vi "Servo.vi"(8 "error in (no error)":errorcluster, 9 "Slow":bool, 10 "Function":T1, 11 "Servo":tag) -> (0 "error out":errorcluster)   [LabVIEW 2014]
uses:
  Controls/Conveyor Belt Functions.ctl
  <vilib>/myRIO/Common/Instrument Driver Framework/myRIO v1.0/PWM/vis/myRIO v1.1 Open PWM.vi
  <vilib>/myRIO/Common/Instrument Driver Framework/Utilities/vis/Validate Channels.vi
  <vilib>/myRIO/Common/Instrument Driver Framework/myRIO v1.0/PWM/vis/myRIO v1.0 Reserve PWM.vi
  <vilib>/myRIO/Common/Instrument Driver Framework/myRIO v1.0/PWM/vis/myRIO v1.0 Build MUX Configuration PWM.vi
  <vilib>/myRIO/Common/Instrument Driver Framework/myRIO v1.0/Resource Manager/vis/myRIO v1.0 Reserve Channel List.vi
  <vilib>/myRIO/Common/Instrument Driver Framework/myRIO v1.0/Resource Manager/vis/myRIO v1.0 Create Configuration List.vi
  <vilib>/myRIO/Common/Instrument Driver Framework/myRIO v1.0/Resource Manager/vis/myRIO v1.0 Reserve Channel.vi
  <vilib>/myRIO/Common/Instrument Driver Framework/myRIO v1.0/Resource Manager/vis/myRIO v1.0 Unreserve Channel.vi
  <vilib>/myRIO/Common/Instrument Driver Framework/myRIO v1.0/Resource Manager/vis/myRIO v1.0 Build Mutex Name.vi
  <vilib>/Utility/VariantDataType/GetNumericInfo.vi
  <vilib>/Utility/error.llb/Error Cluster From Error Code.vi
  <vilib>/myRIO/Common/Instrument Driver Framework/myRIO v1.0/myRIO v1.1 Open.vi
  <vilib>/myRIO/Common/Instrument Driver Framework/Utilities/vis/IO Manager.vi
  <vilib>/myRIO/Common/Instrument Driver Framework/Utilities/vis/Configuration Manager.vi
  <vilib>/myRIO/Common/Instrument Driver Framework/myRIO v1.0/Resource Manager/vis/myRIO v1.0 Configure IO.vi
  <vilib>/myRIO/Common/Instrument Driver Framework/myRIO v1.0/myRIO v1.0 Close.vi
  <vilib>/myRIO/Common/Instrument Driver Framework/myRIO v1.0/PWM/vis/myRIO v1.0 Write PWM.vi
  <vilib>/myRIO/Instrument Drivers/Onboard IO/PWM/PWM.lvlib
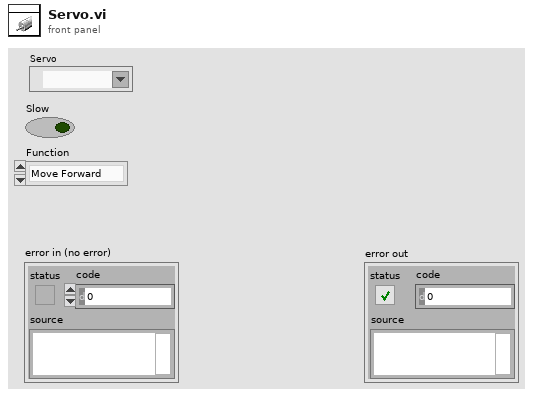
[diagram p1: front panel]
types:
  T1 = typedef "Conveyor Belt Functions.ctl" = enum16{"Move Forward", "Move Backward", "Stop"}
  T2 = typedef "PWM.lvlib/PWM Reference.ctl" = cluster{"myRIO Reference":T3, "PWM Channels Enum":T7, "PWM Configuration":T8}
  T3 = typedef "myRIO Generic Hardware Reference.ctl" = cluster{"myRIO Model":T4, "myRIO Hardware Reference":T5}
  T4 = typedef "Hardware Version Enum.ctl" = enum16{"Unknown", "myRIO-1900", "myRIO-1950"}
  T5 = typedef "myRIO v1.0 Reference.ctl" = cluster{"Generic FPGA Reference":T6, "Allow multiple opens":bool}
  T6 = typedef "Generic FPGA Reference.ctl" = refnum<k20>
  T7 = typedef "PWM Channels Enum.ctl" = enum16{"Not Connected", "C/PWM0", "C/PWM1", "A/PWM0", "A/PWM1", "A/PWM2", "B/PWM0", "B/PWM1", "B/PWM2"}
  T8 = typedef "PWM.lvlib/PWM Configuration.ctl" = cluster{"Frequency":dbl, "Duty Cycle":dbl}
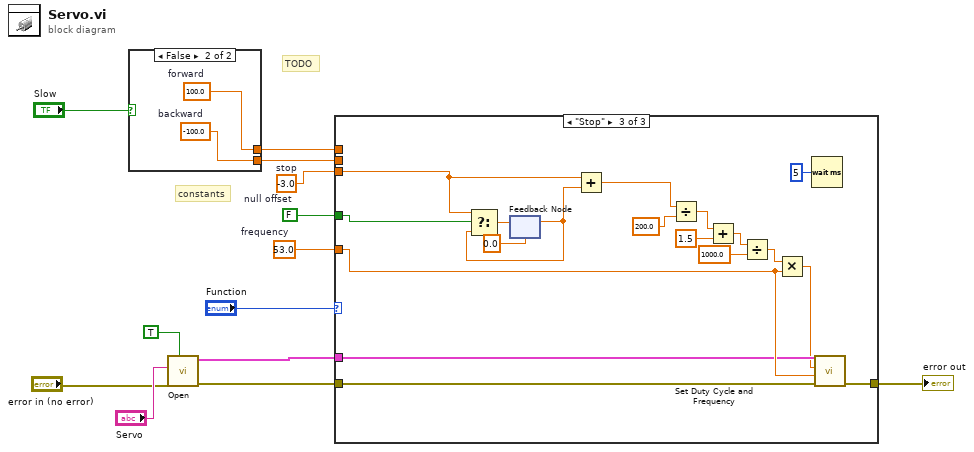
[diagram p0: block diagram]
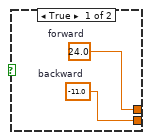
[diagram p2: hidden frame]
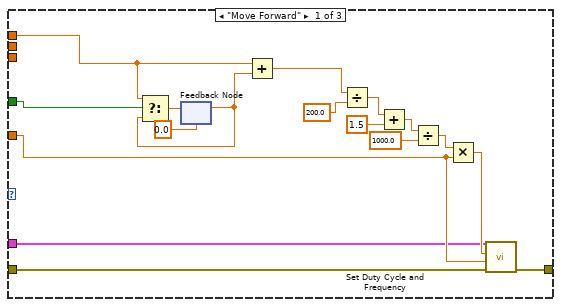
[diagram p3: hidden frame]
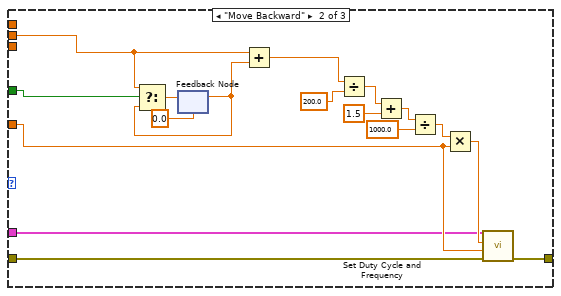
[diagram p4: hidden frame]
diagram:
  w8 = FALSE  # null offset
  w9 = 53.0  # frequency
  w2 = -3.0  # stop
  # "TODO"
  # "constants"
  n1 = case shown="False" "Slow" {
    tunnel: [w15 w17] -> w11
    tunnel: [w14 w16] -> w10
    frame True {
      w15 = -11.0  # backward
      w14 = 24.0  # forward
    }
    frame False {
      w17 = -100.0  # backward
      w16 = 100.0  # forward
    }
  }
  n2 = call <vilib>:"Open.vi"("Allow multiple opens?"=TRUE, "error in (no error)"="error in (no error)", "Channel Name"="Servo") -> ("error out"=w13:errorcluster, "PWM Ref Out"=w7:T2)  [unwired: 7 in]
  n3 = case shown="\"Stop\"" "Function" {
    tunnel: w13 -> [w22 w46 w69]
    tunnel: [w23 w39 w68] -> w6
    tunnel: w7 -> [w18 w35 w65]
    tunnel: w11 -> [_ w38 _]
    tunnel: w10 -> [w21 _ _]
    tunnel: w2 -> [_ _ w52]
    tunnel: w9 -> [w19 w37 w67]
    tunnel: w8 -> [w20 w36 w66]
    frame "Move Forward" {
      n4 = feedback #1(0.0 ("position [%FS]")) -> (w31:dbl)
      n5 = Select(t=w21, s=w20, f=w31) -> (s? t:f=w29:dbl)
      n6 = feedback-in #1(w29) -> ()
      n7 = Add(x=w21, y=w31) -> (x+y=w30:dbl)
      n8 = Divide(x=w30, y=200.0) -> (x/y=w25:dbl)
      n9 = Add(x=w25, y=1.5) -> (x+y=w27:dbl)
      n10 = Divide(x=w27, y=1000.0) -> (x/y=w32:dbl)
      n11 = Multiply(x=w32, y=w19) -> (x*y=w33:dbl)
      n12 = call <vilib>:"Set Duty Cycle and Frequency.vi"("error in (no error)"=w22, "Frequency [Hz]"=w19, "Duty Cycle"=w33, "PWM Ref In"=w18) -> ("error out"=w23:errorcluster)  [unwired: 5 in, 1 out]
    }
    frame "Move Backward" {
      n13 = feedback #2(0.0 ("position [%FS]")) -> (w43:dbl)
      n14 = Select(t=w38, s=w36, f=w43) -> (s? t:f=w45:dbl)
      n15 = feedback-in #2(w45) -> ()
      n16 = Add(x=w38, y=w43) -> (x+y=w44:dbl)
      n17 = Divide(x=w44, y=200.0) -> (x/y=w50:dbl)
      n18 = Add(x=w50, y=1.5) -> (x+y=w48:dbl)
      n19 = Divide(x=w48, y=1000.0) -> (x/y=w42:dbl)
      n20 = Multiply(x=w42, y=w37) -> (x*y=w41:dbl)
      n21 = call <vilib>:"Set Duty Cycle and Frequency.vi"("error in (no error)"=w46, "Frequency [Hz]"=w37, "Duty Cycle"=w41, "PWM Ref In"=w35) -> ("error out"=w39:errorcluster)  [unwired: 5 in, 1 out]
    }
    frame "Stop" {
      n22 = feedback #3(0.0 ("position [%FS]")) -> (w61:dbl)
      n23 = Select(t=w52, s=w66, f=w61) -> (s? t:f=w59:dbl)
      n24 = feedback-in #3(w59) -> ()
      n25 = Add(x=w52, y=w61) -> (x+y=w60:dbl)
      n26 = Divide(x=w60, y=200.0) -> (x/y=w55:dbl)
      n27 = Add(x=w55, y=1.5) -> (x+y=w57:dbl)
      n28 = Divide(x=w57, y=1000.0) -> (x/y=w62:dbl)
      n29 = Multiply(x=w62, y=w67) -> (x*y=w63:dbl)
      n30 = Wait (ms)(milliseconds to wait=u32 5) -> ()  [unwired: 1 out]
      n31 = call <vilib>:"Set Duty Cycle and Frequency.vi"("error in (no error)"=w69, "Frequency [Hz]"=w67, "Duty Cycle"=w63, "PWM Ref In"=w65) -> ("error out"=w68:errorcluster)  [unwired: 5 in, 1 out]
    }
  }
  "error out" <- w6
